vi "change path.vi"(10 "string":string, 11 "path":path) -> (3 "appended path":path)   [LabVIEW 2020, in "ThorlabsWavefrontDS.lvclass"]
uses:
  ThorlabsWavefrontDS.lvclass
panel:
  in  "string":string
  out "appended path":path
  in  "Path":path
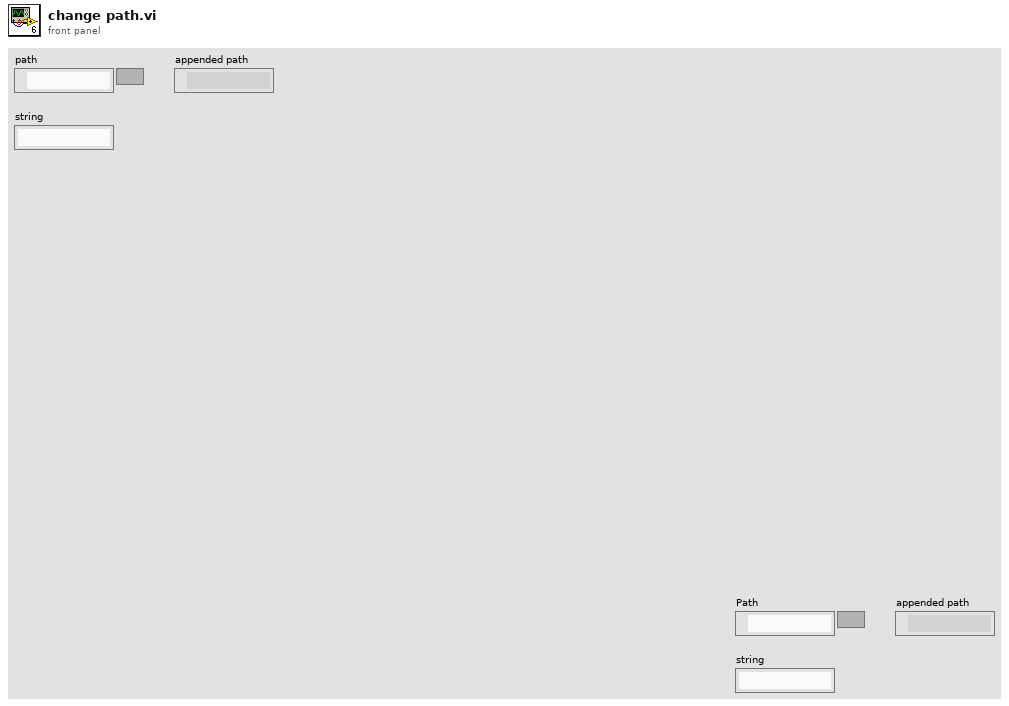
[diagram p1: front panel]
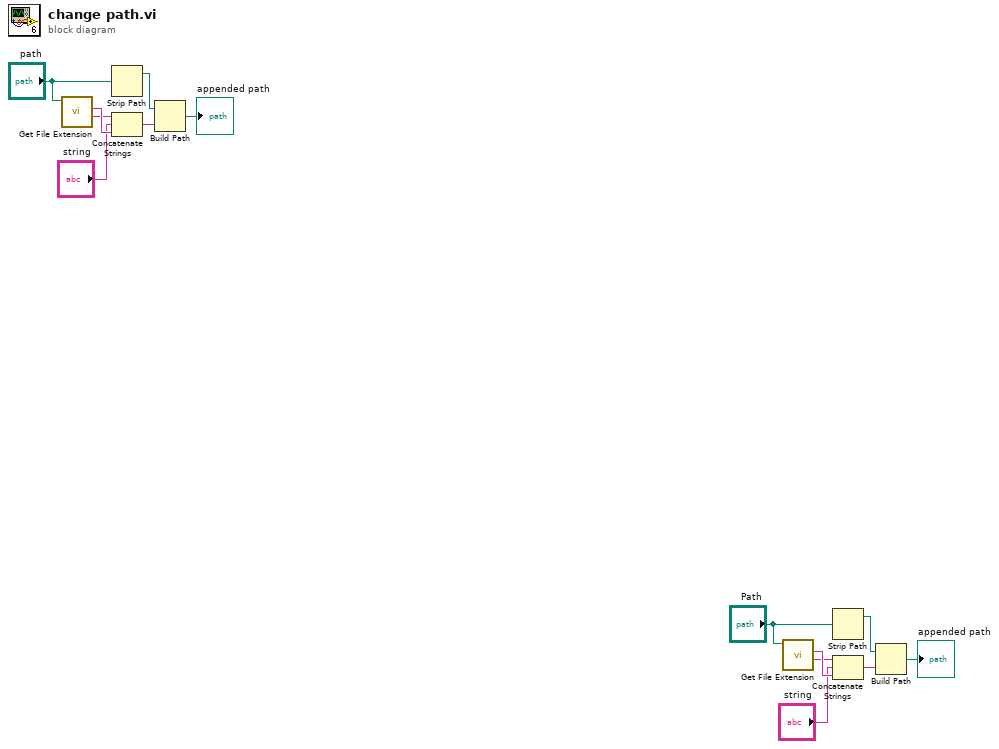
[diagram p0: block diagram]
diagram:
  n1 = call <vilib>:"Get File Extension.vi"("file"="path") -> ("filename without extension"=w2:string, "lowercase file extension"=w3:string)  [unwired: 6 in, 3 out]
  n2 = Strip Path(path="path") -> (stripped path=w5:path)  [unwired: 1 out]
  n3 = Concatenate Strings(w2, "string", w3) -> (w4:string)
  n4 = Build Path(base path=w5, name or relative path=w4) -> (appended path=→"appended path":path)
  n5 = call <vilib>:"Get File Extension.vi"("file"="Path") -> ("filename without extension"=w9:string, "lowercase file extension"=w10:string)  [unwired: 6 in, 3 out]
  n6 = Strip Path(path="Path") -> (stripped path=w12:path)  [unwired: 1 out]
  n7 = Concatenate Strings(w9, "string", w10) -> (w11:string)
  n8 = Build Path(base path=w12, name or relative path=w11) -> (appended path=→"appended path":path)
